vi "ActionVIOnSave.vi"(8 "error in (no error)":errorcluster, 11 "Device Item Ref in":T1 format="%.0x") -> (0 "error out":errorcluster, 3 "Device Item Ref out":T1 format="%.0x")   [LabVIEW 2020, in "DSF System Explorer.lvlib"]
uses:
  DSF System Explorer.lvlib
  <vilib>/NI VeriStand/Custom Device API/Custom Device Item Ref.ctl
  <vilib>/NI VeriStand/Custom Device API/Custom Device API.lvlib
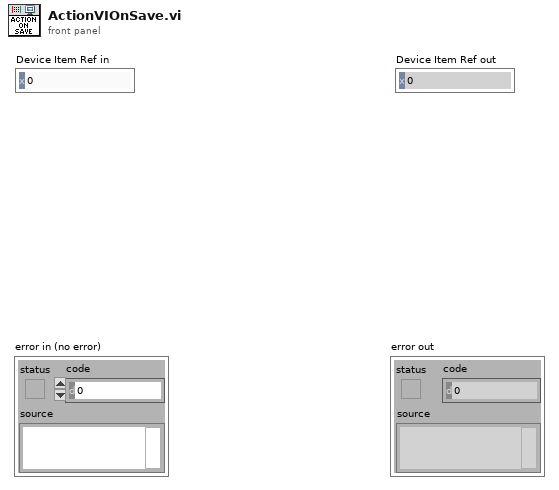
[diagram p1: front panel]
types:
  T1 = typedef "Custom Device API.lvlib/Custom Device Item Ref.ctl" = u64
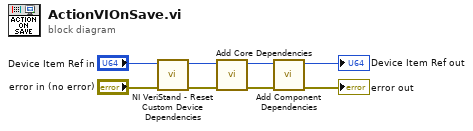
[diagram p0: block diagram]
diagram:
  n1 = call <vilib>:"NI VeriStand - Reset Custom Device Dependencies.vi"("error in (no error)"="error in (no error)", "Device Ref in"="Device Item Ref in") -> ("error out"=w5:errorcluster, "Device Ref out"=w6:T1)  [unwired: 8 in]
  n2 = call "Add Core Dependencies.vi"("error in (no error)"=w5, "Item Ref in"=w6) -> ("error out"=w1:errorcluster, "Device Ref out"=w2:T1)  [unwired: 8 in]
  n3 = call "Add Component Dependencies.vi"("error in (no error)"=w1, "Device Item Ref in"=w2) -> ("error out"=→"error out":errorcluster, "Device Ref out"=→"Device Item Ref out":T1)  [unwired: 7 in, 1 out]
